vi "Reset Tag.vi"(8 "error in (no error)":errorcluster, 9 "New Tag":string, 10 "Original Tag":string, 11 "Tree in":refnum<class "Tree.lvclass">) -> (0 "error out":errorcluster, 3 "Tree out":refnum<class "Tree.lvclass">)   [LabVIEW 2024, in "Tree.lvclass"]
uses:
  Tree.lvclass
  Tree.lvclass/Tree.ctl
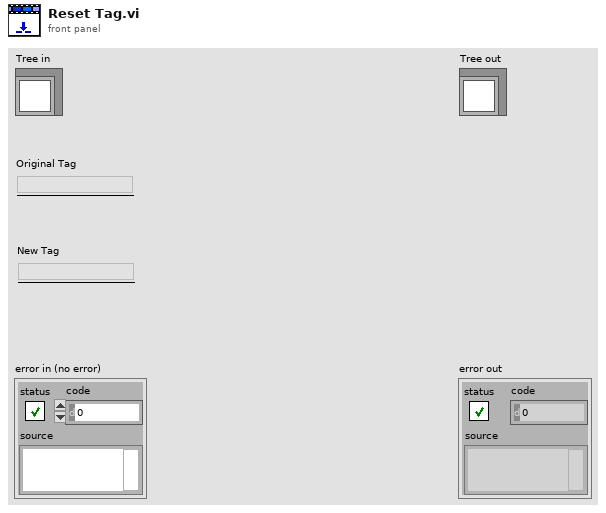
[diagram p1: front panel]
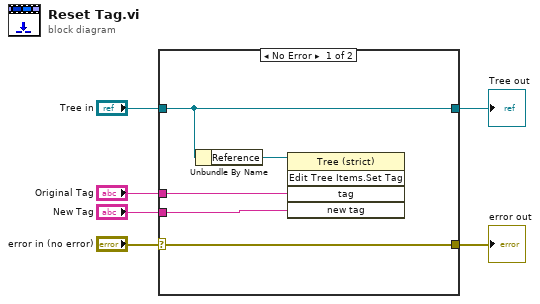
[diagram p0: block diagram]
diagram:
  n1 = case shown="No Error" "error in (no error)" {
    selector: "error in (no error)" -> [w11 w13]
    tunnel: [w11 w13] -> w5
    tunnel: [w10 w12] -> w3
    tunnel: "Tree in" -> [w10 w12]
    tunnel: "Original Tag" -> [w8 _]
    tunnel: "New Tag" -> [w7 _]
    frame No Error {
      n2 = Unbundle By Name(w10) -> ("Reference"=w9:refnum<vi>)
      n3 = invoke class="Tree (strict)" method="Edit Tree Items.Set Tag"(reference=w9, "tag"=w8, "new tag"=w7) -> ()  [unwired: 2 in, 5 out]
    }
    frame Error {
    }
  }
  "error out" <- w5
  "Tree out" <- w3
